vi "Init.vi"(8 "error in (no error)":errorcluster, 11 "DtoA in":refnum<class "Gage 300MHz.lvclass">) -> (0 "error out":errorcluster, 3 "DtoA out":refnum<class "Gage 300MHz.lvclass">)   [LabVIEW 2014, in "Gage 300MHz.lvclass"]
uses:
  Gage 300MHz.lvclass
  External Clock.lvclass
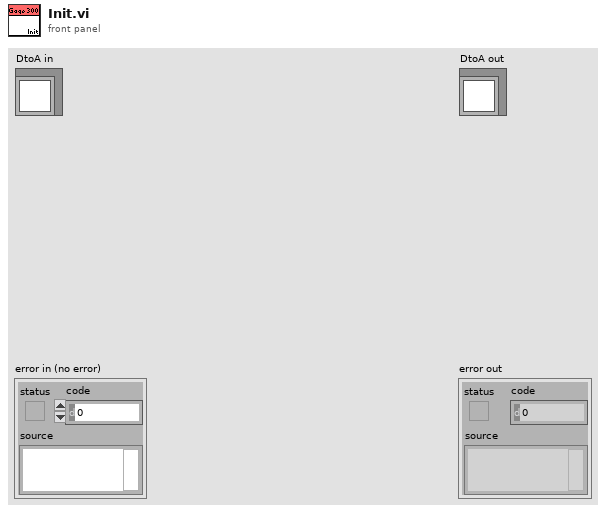
[diagram p1: front panel]
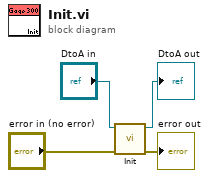
[diagram p0: block diagram]
diagram:
  n1 = call-parent "Init.vi"("error in (no error)"="error in (no error)", "DtoA in"="DtoA in") -> ("error out"=→"error out":errorcluster, "DtoA out"=→"DtoA out":refnum<class "Gage 300MHz.lvclass">)  [unwired: 8 in]
